vi "test (子VI).vi"() -> (3 "XY图":cluster{"X":dbl, "Y":dbl}[](graph))   [LabVIEW 2019]
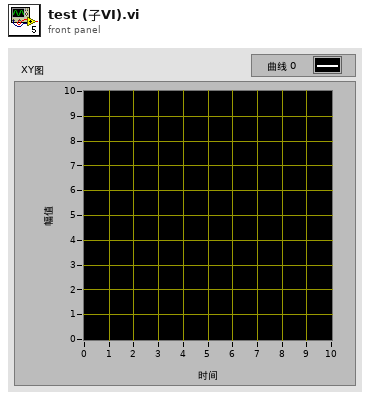
[diagram p1: front panel]
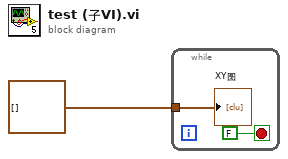
[diagram p0: block diagram]
diagram:
  n1 = while {
    tunnel: cluster{"X":dbl, "Y":dbl}[] [] ("XY图") -> [w3]
    stop <- FALSE stop-if-true
    "XY图" <- w3
  }
